vi "Save Background Img.vi"(9 "Acq Img":T3, 11 "CamConfigCluster":T2={"ID"=0.0, "Name"="", "DeviceID"={"Slot Connector"=0, "IP Adress"="", "Port"=0, "Type"=""}, "CorrectConfig Cluster"={"Detection Parameters"={"Contrast"=0, "Treshold"=0, "Max Intensity"=0, "Max Intensity%"=0, "Rx"=0, "Ry"=0, "R%"=0.0}, "Reverse"={"Reverse X"=FALSE, "Reverse Y"=FALSE}, "Target"={"X Target"=0.0, "Y Target"=0.0}, "Region of Interest"=[-1, -1, 32000, 32000], "Correction Parameters"={"X"=5.0, "Y"=5.0, "Movement Type"=0}, "Acquisition Parameters"={"Brightness"=0.0, "Contrast"=1.0, "Saturation"=1.0, "White level"=0.7}, "Background Path"=path "", "Reference Path"=path "", "XCalibration"=[], "YCalibration"=[]}, "Ontrak Channel"=0, "IMAQdx Session 2"="cam2", "ImageServer"={"IPAddress"="", "Port"=0}} {"CorrectConfig Cluster"."Acquisition Parameters"."White level" scale=0.3..1.26 scale format="%#_2f"; "CorrectConfig Cluster"."Acquisition Parameters"."Saturation" scale=0.5..1.5 scale format="%#_3f"; "CorrectConfig Cluster"."Acquisition Parameters"."Contrast" scale=0.4..1.5 scale format="%#_3f"; "CorrectConfig Cluster"."Acquisition Parameters"."Brightness" scale=-50.0..50.0 scale format="%#_2f"; "CorrectConfig Cluster"."Correction Parameters"."Movement Type" items=["Step", "Proportionnal"]; "CorrectConfig Cluster"."Target"."X Target" format="%#_5g"; "CorrectConfig Cluster"."Target"."Y Target" format="%#_5g"; "CorrectConfig Cluster"."Detection Parameters"."Max Intensity%" max=100 step=1}) -> (3 "Background Path":path)   [LabVIEW 2013]
uses:
  <vilib>/vision/Image Controls.llb/IMAQ Image.ctl
  <vilib>/userdefined/High Color/IMAQdx.ctl
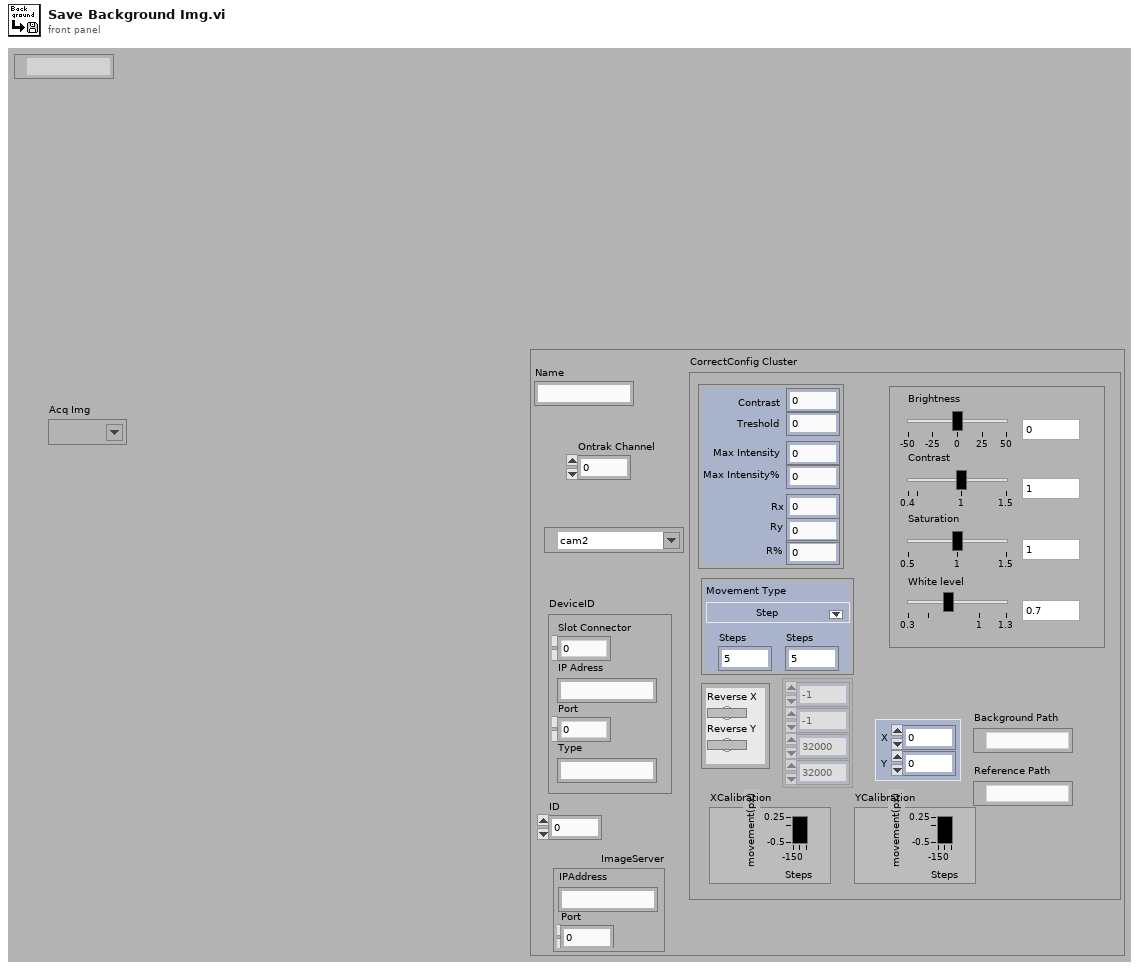
[diagram p1: front panel]
types:
  T1 = typedef "IMAQdx.ctl" = refnum<k21>
  T2 = cluster{"ID":dbl, "Name":string, "DeviceID":cluster{"Slot Connector":i32, "IP Adress":string, "Port":i32, "Type":string}, "CorrectConfig Cluster":cluster{"Detection Parameters":cluster{"Contrast":i32, "Treshold":u8, "Max Intensity":i32, "Max Intensity%":u8, "Rx":i32, "Ry":i32, "R%":sgl}, "Reverse":cluster{"Reverse X":bool, "Reverse Y":bool}, "Target":cluster{"X Target":sgl, "Y Target":sgl}, "Region of Interest":i32[], "Correction Parameters":cluster{"X":sgl, "Y":sgl, "Movement Type":u16}, "Acquisition Parameters":cluster{"Brightness":dbl, "Contrast":dbl, "Saturation":dbl, "White level":dbl}, "Background Path":path, "Reference Path":path, "XCalibration":cluster{dbl, dbl}[], "YCalibration":cluster{dbl, dbl}[]}, "Ontrak Channel":i16, "IMAQdx Session 2":T1, "ImageServer":cluster{"IPAddress":string, "Port":i32}}
  T3 = typedef "IMAQ Image.ctl" = refnum<image>
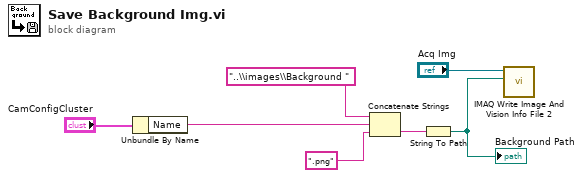
[diagram p0: block diagram]
diagram:
  n1 = Unbundle By Name("CamConfigCluster") -> ("Name"=w3:string)
  n2 = Concatenate Strings("..\\images\\Background ", w3, ".png") -> (w6:string)
  n3 = String To Path(string=w6) -> (path=w5:path)
  "Background Path" <- w5
  n4 = call "IMAQ Write Image And Vision Info File 2"("File Path"=w5, "Image"="Acq Img") -> ()  [unwired: 8 in, 2 out]
